vi "Save_to_Project.vi"(8 "error in (no error)":errorcluster, 9 "index in":string, 10 "buildObject":T1, 11 "Class in":refnum<class "IB_CtrFile.lvclass">) -> (0 "error out":errorcluster, 1 "index out":string, 2 "buildObject out":T1, 3 "Class out":refnum<class "IB_CtrFile.lvclass">, 5 "saved?":bool)   [LabVIEW 2020, in "IB_CtrFile.lvclass"]
uses:
  <vilib>/AppBuilder/IB_Classes/Source/File/CtrFile/IB_CtrFile.lvclass
  <vilib>/AppBuilder/IB_Classes/Source/File/CtrFile/IB_CtrFile.lvclass/IB_CtrFile.ctl
  <vilib>/AppBuilder/IB_Classes/Source/File/IB_Source_File.lvclass
  e:/builds/penguin/labview/branches/2020/dev/dist/vi.lib/AppBuilder/IB_Classes/Source/File/IB_Source_File.lvclass
  e:/builds/penguin/labview/branches/2020/dev/dist/vi.lib/AppBuilder/IB_Classes/Source/IB_Source.lvclass
  e:/builds/penguin/labview/branches/2020/dev/dist/vi.lib/AppBuilder/IB_Classes/Source/File/CtrFile/IB_CtrFile.lvclass
  <resource>/Framework/Providers/API/ItemRef.ctl
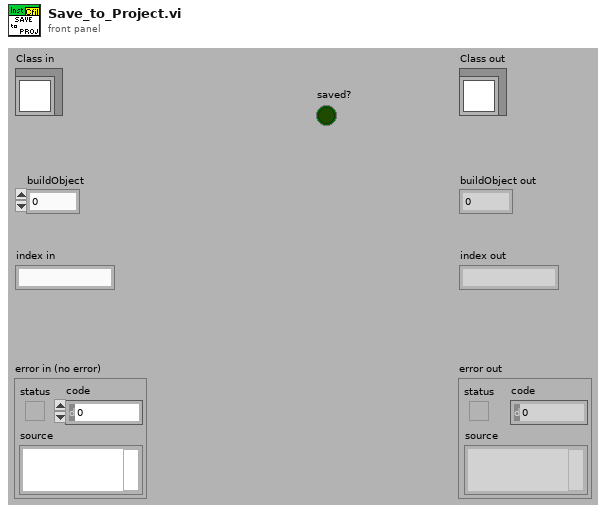
[diagram p1: front panel]
types:
  T1 = typedef "ItemRef.ctl" = u64
  T2 = typedef "IB_Source_File.ctl" = cluster{"Attributes":i16, "RegCOM":bool, "unlock":bool, "shortcuts":refnum<class "IB_Shortcut.lvclass">[], "EXE_install":bool, "CmdArg_install":string, "EXE_uninstall":bool, "CmdArg_uninstall":string}
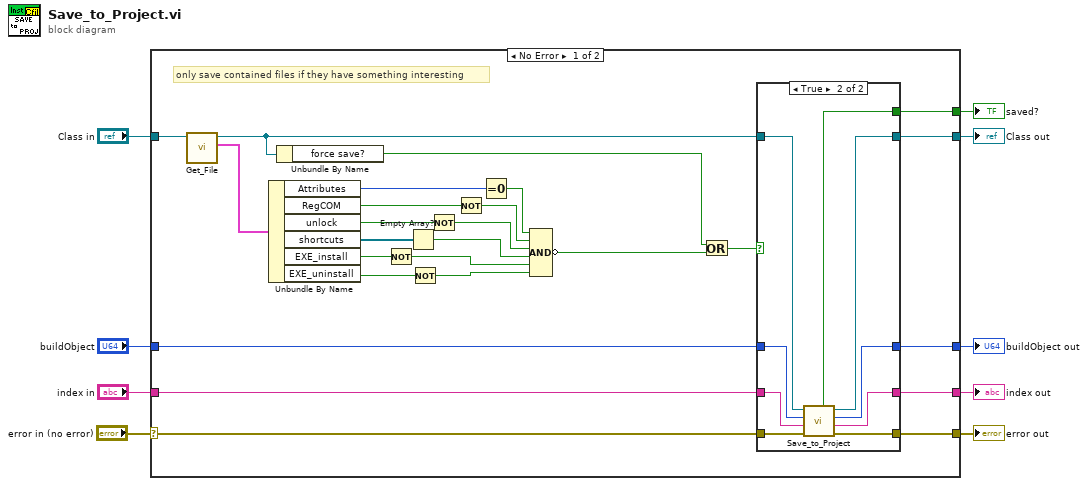
[diagram p0: block diagram]
diagram:
  n1 = case shown="No Error" "error in (no error)" {
    selector: "error in (no error)" -> [w29 w52]
    tunnel: [w35 w52] -> w9
    tunnel: [w34 w51] -> w8
    tunnel: [w33 w50] -> w7
    tunnel: [w32 w49] -> w6
    tunnel: "index in" -> [w31 w51]
    tunnel: "buildObject" -> [w30 w50]
    tunnel: "Class in" -> [w27 w49]
    tunnel: [w28 _] -> w1
    frame No Error {
      # "only save contained files if they have something interesting"
      n2 = call <vilib>:"Get_File.vi"("IB_Source_File in"=w27) -> ("data"=w26:T2, "IB_Source_File out"=w15:refnum<class "IB_CtrFile.lvclass">)  [unwired: 1 in, 8 out]
      n3 = Unbundle By Name(w26) -> ("Attributes"=w24:i16, "RegCOM"=w21:bool, "unlock"=w19:bool, "shortcuts"=w25:refnum<class "IB_Shortcut.lvclass">[], "EXE_install"=w17:bool, "EXE_uninstall"=w11:bool)
      n4 = Unbundle By Name(w15) -> ("force save?"=w14:bool)
      n5 = Not(x=w17) -> (.not. x?=w16:bool)
      n6 = Empty Array?(array=w25) -> (empty?=w23:bool)
      n7 = Not(x=w11) -> (.not. x?=w10:bool)
      n8 = Not(x=w19) -> (.not. x?=w18:bool)
      n9 = Not(x=w21) -> (.not. x?=w20:bool)
      n10 = Equal To 0?(x=w24) -> (x = 0?=w22:bool)
      n11 = Compound Arithmetic op=AND(w22, w20, w18, w23, w16, w10) -> (invert w13:bool)
      n12 = Or(x=w14, y=w13) -> (x .or. y?=w12:bool)
      n13 = case shown="True" w12 {
        tunnel: [w39 w48] -> w35
        tunnel: [w38 w47] -> w34
        tunnel: [w37 w46] -> w33
        tunnel: [w36 w45] -> w32
        tunnel: w31 -> [w38 w44]
        tunnel: w30 -> [w37 w43]
        tunnel: w15 -> [w36 w42]
        tunnel: w29 -> [w39 w41]
        tunnel: [_ w40] -> w28
        frame False {
        }
        frame True {
          n14 = call-parent "Save_to_Project.vi"("error in (no error)"=w41, "index in"=w44, "buildObject"=w43, "Class in"=w42) -> ("error out"=w48:errorcluster, "index out"=w47:string, "buildObject out"=w46:T1, "Class out"=w45:refnum<class "IB_CtrFile.lvclass">, "saved?"=w40:bool)  [unwired: 3 out]
        }
      }
    }
    frame Error {
    }
  }
  "error out" <- w9
  "Class out" <- w6
  "buildObject out" <- w7
  "index out" <- w8
  "saved?" <- w1
